vi "Camera_control_v5.vi"() -> ()   [LabVIEW 2018]
uses:
  C:/Program Files/National Instruments/LabVIEW 2018/uc480DotNet.dll
  uc480DotNet.dll
  <vilib>/MakerHub/LINX/Public/Peripherals/PWM/PWM Set Duty Cycle 1 Chan.vi
  <vilib>/MakerHub/LINX/Public/Utilities/Open Serial.vi
  <vilib>/MakerHub/LINX/Public/Peripherals/PWM/PWM Set Duty Cycle N Chans.vi
  System.Windows.Forms
  <vilib>/MakerHub/LINX/LMH-LINX.lvlib
panel:
  in  "Lamp After On (seconds)":dbl=0.5
  in  "Lamp Prior On (seconds)":dbl=0.5
  in  "Analogue out (PWM) Channel":u8=3
  in  "Serial Port":refnum<visa-resource-name>
  out "Time Stamp 5":timestamp format="%<%H:%M:%S\n%Y/%m/%d>T"
  out "Time Stamp 2":timestamp format="%<%H:%M:%S\n%Y/%m/%d>T"
  out "Boolean":bool
  out "?":u8(slide) scale=0.0..1.0
  in  "Capture Period (hours) 2":dbl=0.005
  in  "stop":bool
  out "Image":picture
  in  "Capture Frequency (minutes)":dbl=0.5
  out "Time Stamp":timestamp format="%<%H:%M:%S\n%Y/%m/%d>T"
  in  "Name of Operator":string="AT"
  in  "Parent Folder":path=path "D:/Dropbox (MIT)/Buonassisi-Group/AMD Team/Campaign 2.0/Degradation"
  in  "Zoom":u16(ring)=1 items=["4X"=4, "2X"=2, "1X"=1]
  in  "PictureBox":refnum<k24>(container)
  out "Serial Number 2":string
  out "Height 2":i32=8
  out "Width 2":i32=8
  out "Bits/Pixel 2":i32=8
  in  "Camera ID":i32
  out "Serial Number":string
  out "Height":i32=8
  out "Width":i32=8
  out "Bits/Pixel":i32=8
  in  "Pixelclock":i32(slide)=33 min=5 max=40 step=1 scale=5.0..40.0
  in  "Framerate":dbl(slide)=33.21525 min=0.47411700449083627 max=15.001275108384213 step=0.014032998230479876 scale=0.47411700449083627..15.001275108384213 scale format="%#.3g"
  in  "Exposure":dbl(slide)=33.21525 min=0.06241666666666667 max=99.86666666666667 step=0.06241666666666667 scale=0.06241666666666667..99.86666666666667 scale format="%#.3g"
  out "Error Out":errorcluster caption="error"
  in  "Load Parameter":bool
  in  "Exit Camera":bool
  in  "Stop Live":bool
  in  "Start Live":bool
  in  "Init Camera":bool
  # "Lamp Control via Arduino (LINX).\n\nSet-up Instructions\n1. Click Tools-->MakerHub-->LINX-->LINX Firmware Wizard\n2. Select Arduino type-->Next\n3. Select the COM Port associated with Arduino.\n    (can be found clicking 'Refresh' from the dropdown)-->Next\n4. Click Next\n5. Click Finish"
  # "Select the COM Port"
  # "Select the Arduino PWM pin\nto which the lamp is connected"
  # "Time for lamp to stablize before each run of photo taking"
  # "Time for lamp to stay on after each run of photo taking"
  # "This is not functional!!! Needs debugging"
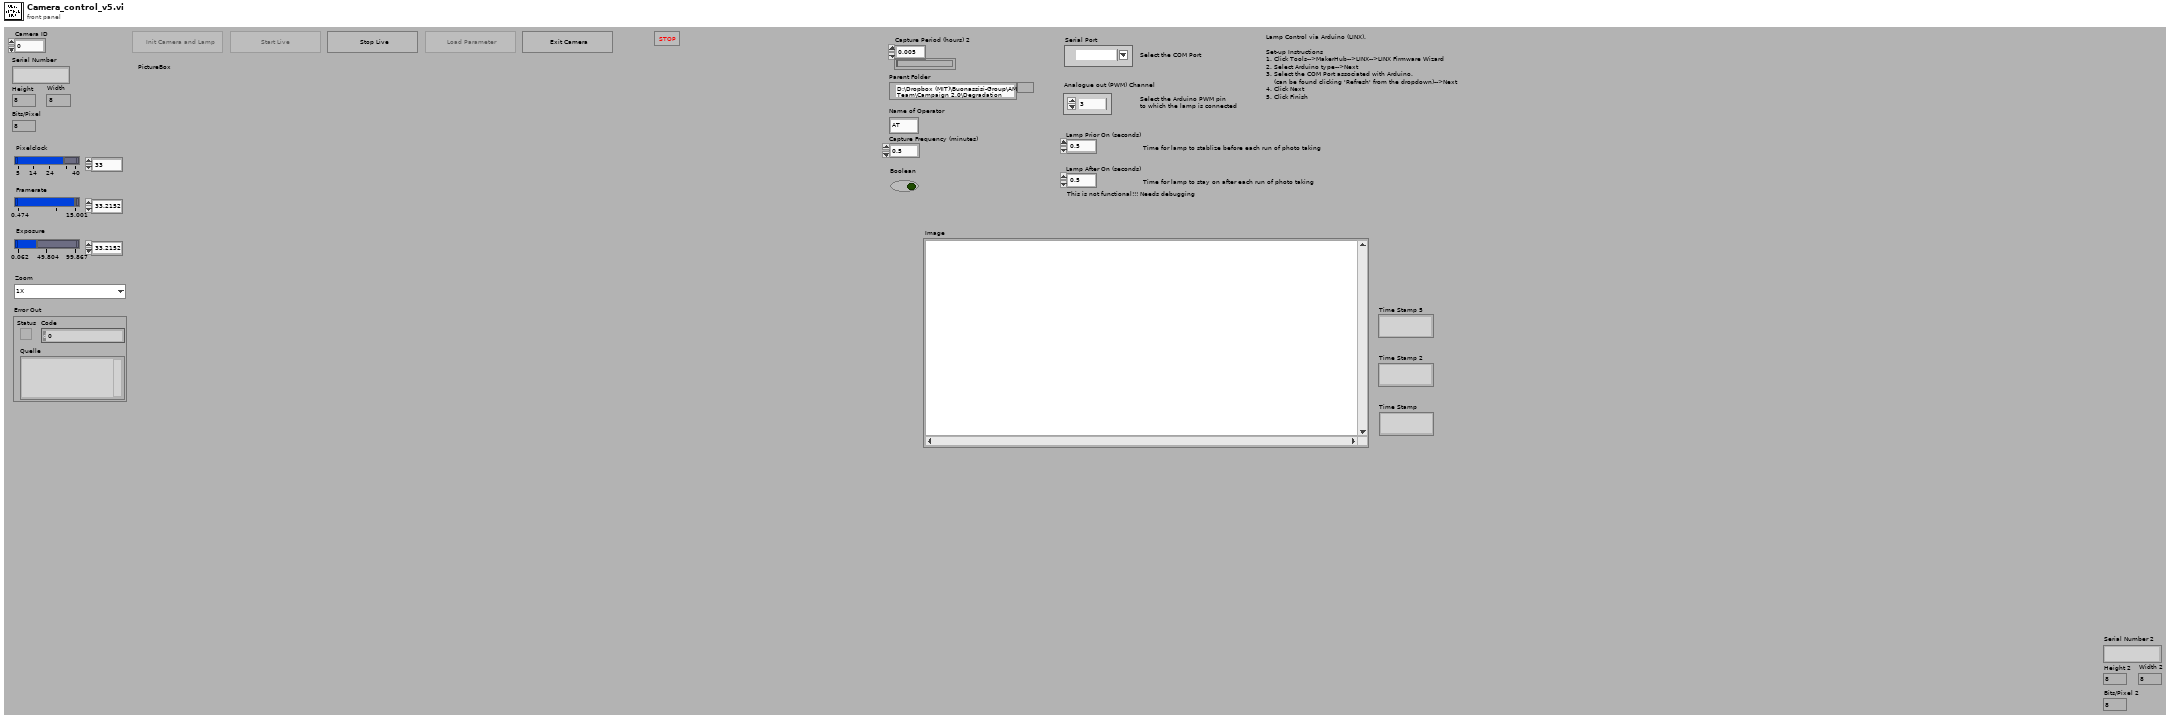
[diagram p1: front panel]
types:
  T1 = typedef "LMH-LINX.lvlib/LINX Ref.ctl" = cluster{"IO":T2, "Interface":T3, "LINX Device Config":T4}
  T2 = typedef "LMH-LINX.lvlib/Platform.ctl" = enum16{"Remote", "Local"}
  T3 = typedef "LMH-LINX.lvlib/Interface.ctl" = enum16{"Serial", "TCP"}
  T4 = typedef "LMH-LINX.lvlib/Device.lvlib/LINX Device Config.ctl" = cluster{"Interface":T3, "COM Port":refnum<visa-resource-name>, "TCP Configuration":T5, "Device Family":u8, "Device ID":u8, "Device Name":string, "TCP Ref":refnum<k5>, "Channels":T6}
  T5 = typedef "LMH-LINX.lvlib/Device.lvlib/TCP Config.ctl" = cluster{"IP Address":string, "Port":u16}
  T6 = typedef "LMH-LINX.lvlib/Channels.ctl" = cluster{"DI":u8[], "DO":u8[], "AI":u8[], "AO":u8[], "PWM":u8[], "QE":u8[], "UART":u8[], "I2C 2":u8[], "SPI":u8[], "CAN":u8[], "Servo":u8[], "AI Ref (V)":dbl, "AI Resolution (Bits)":u8, "AO Ref (V)":dbl, "AO Resolution (Bits)":u8}
  T7 = enum8{"Enabled", "Disabled", "Disabled and Grayed Out"}
  T8 = typedef "imagedata.ctl" = cluster{"image type":i32, "image depth":i32, "image":u8[], "mask":u8[], "colors":u32[], "Rectangle":cluster{"left":i16, "top":i16, "right":i16, "bottom":i16}}
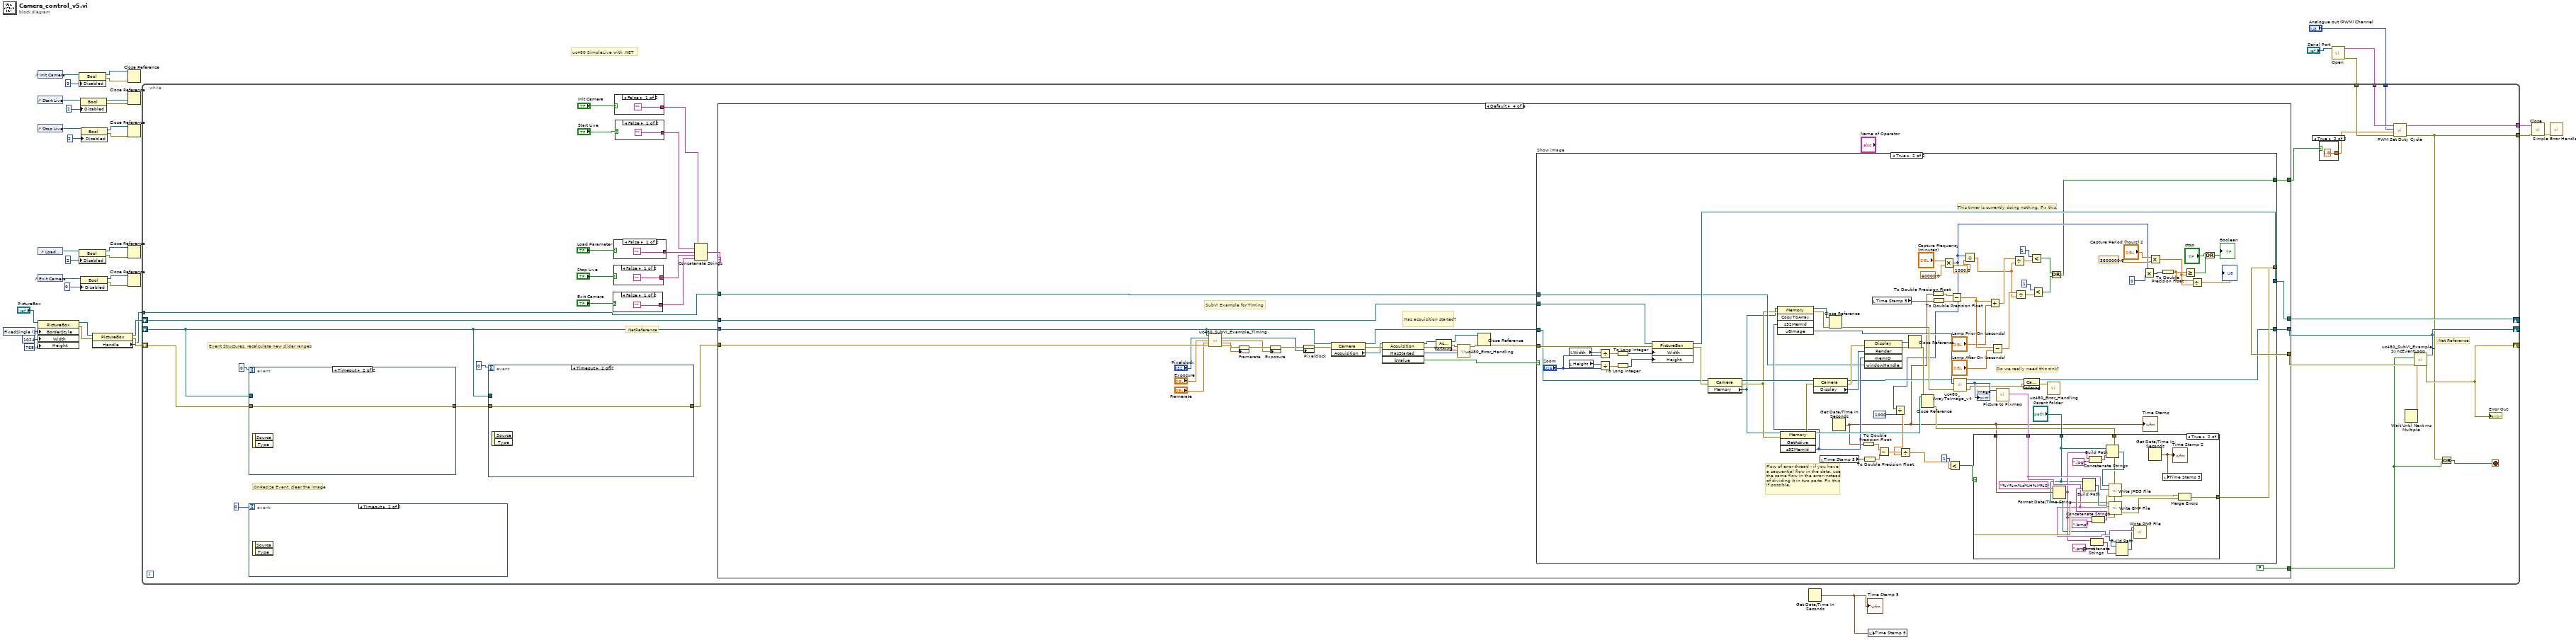
[diagram p0: block diagram]
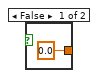
[diagram p2: hidden frame]
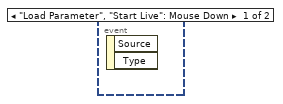
[diagram p3: hidden frame]
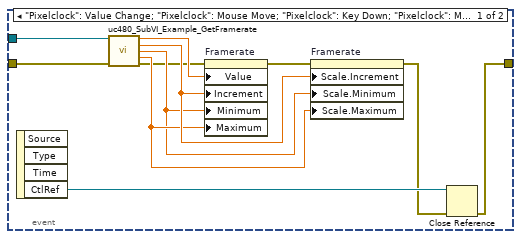
[diagram p4: hidden frame]
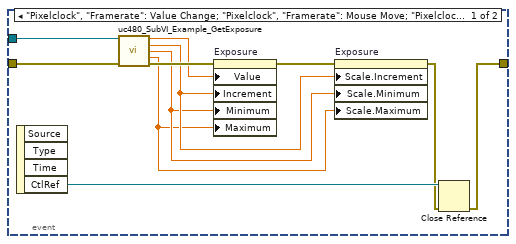
[diagram p5: hidden frame]
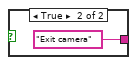
[diagram p6: hidden frame]
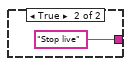
[diagram p7: hidden frame]
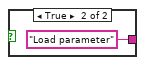
[diagram p8: hidden frame]
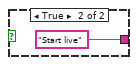
[diagram p9: hidden frame]
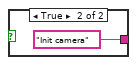
[diagram p10: hidden frame]
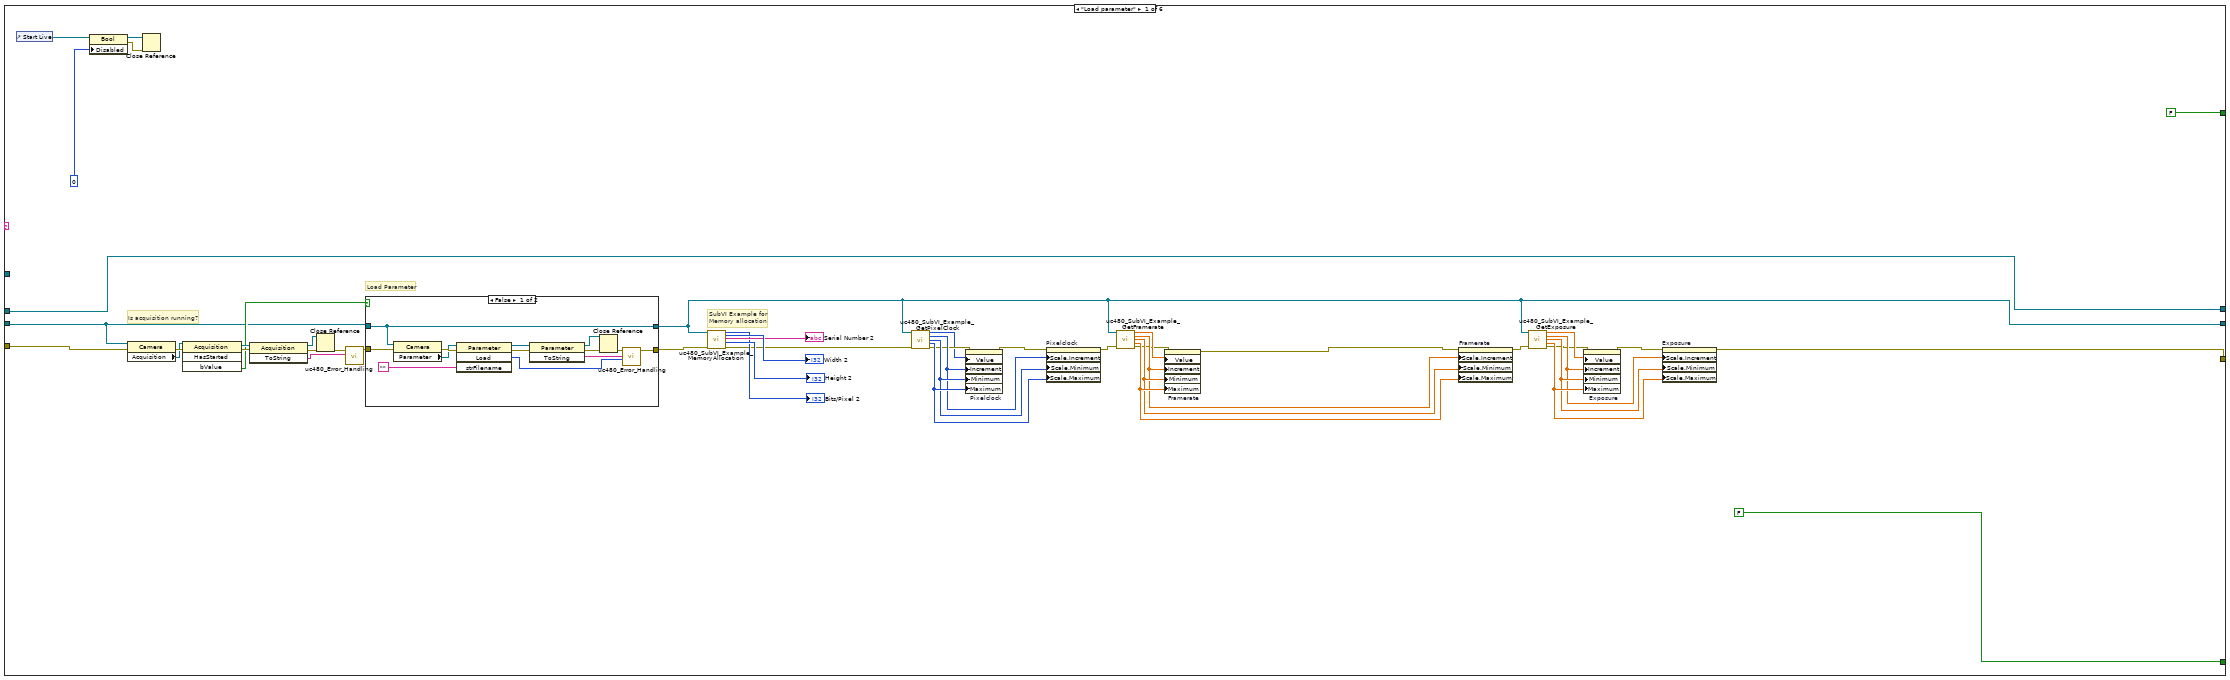
[diagram p11: hidden frame]
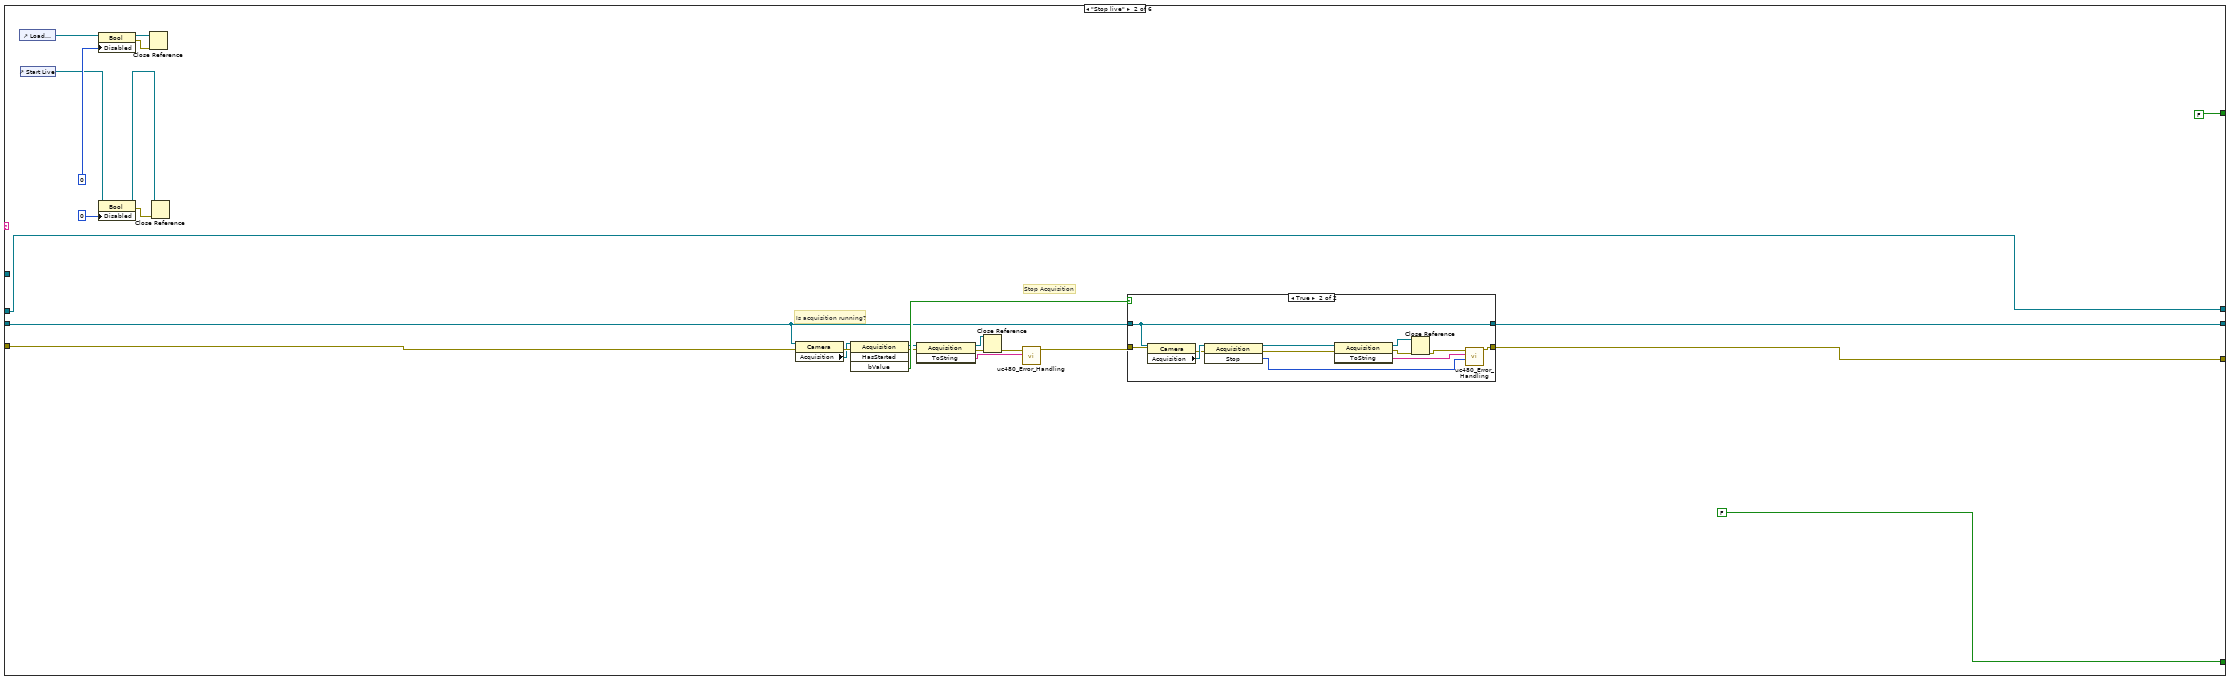
[diagram p13: hidden frame]
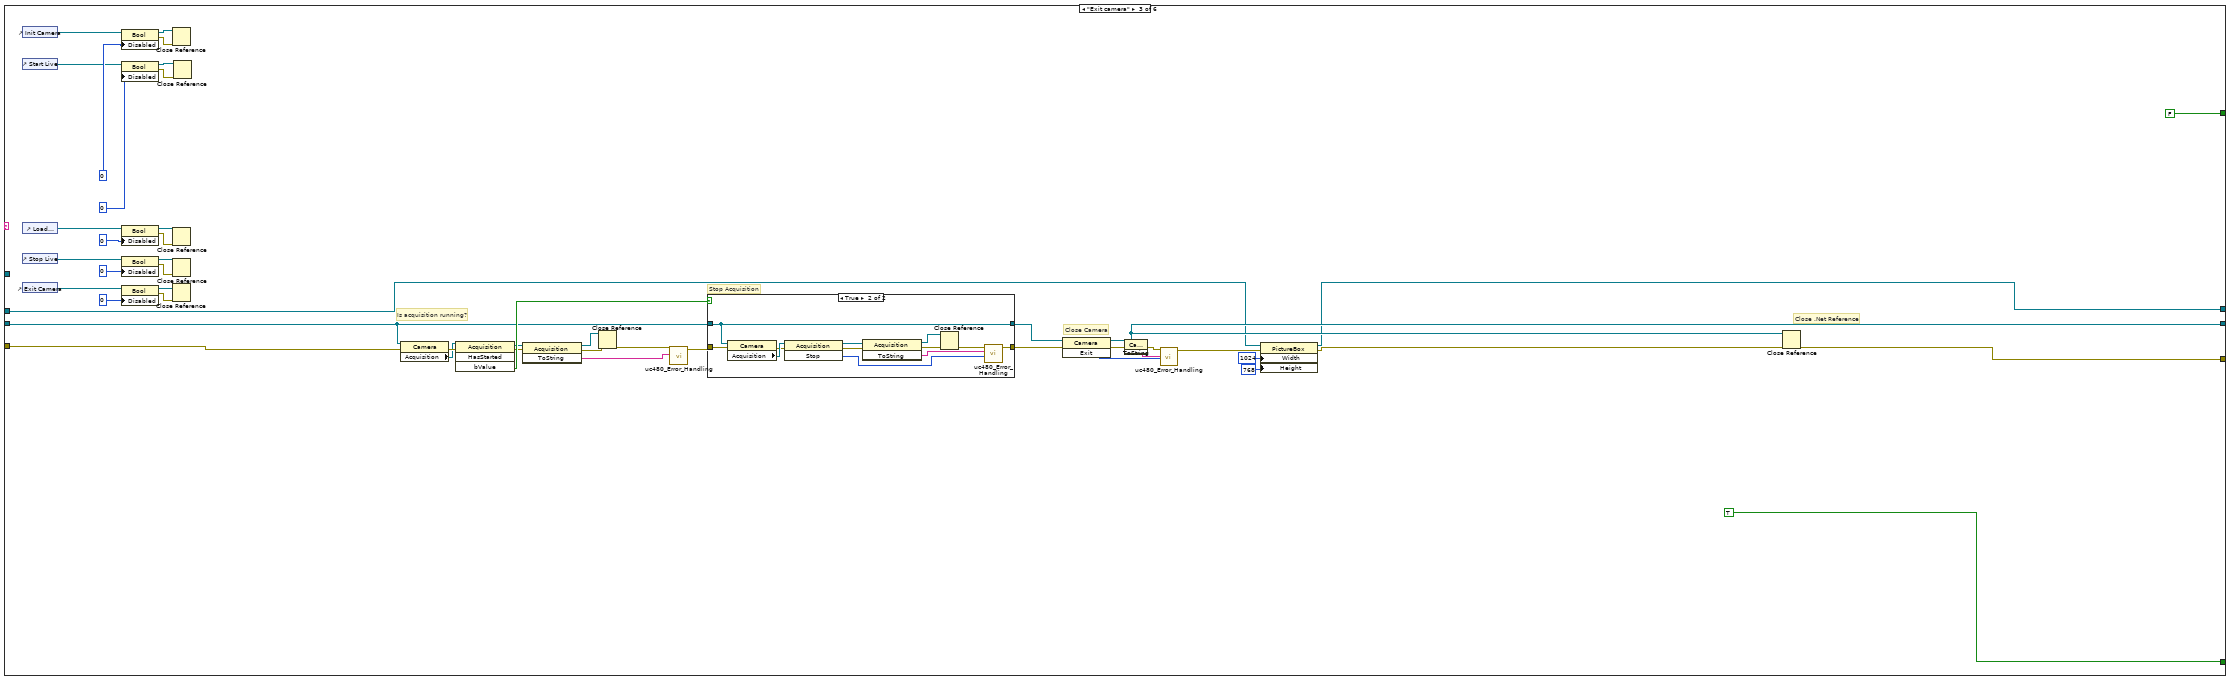
[diagram p15: hidden frame]
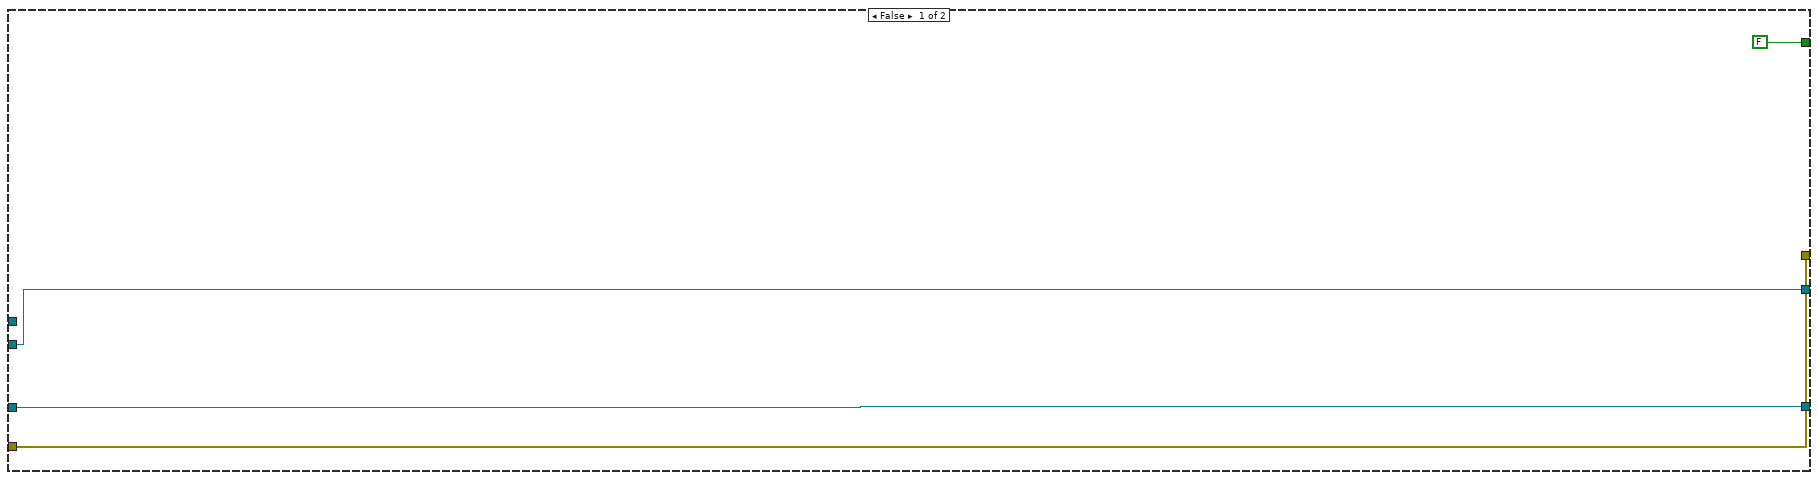
[diagram p17: hidden frame]
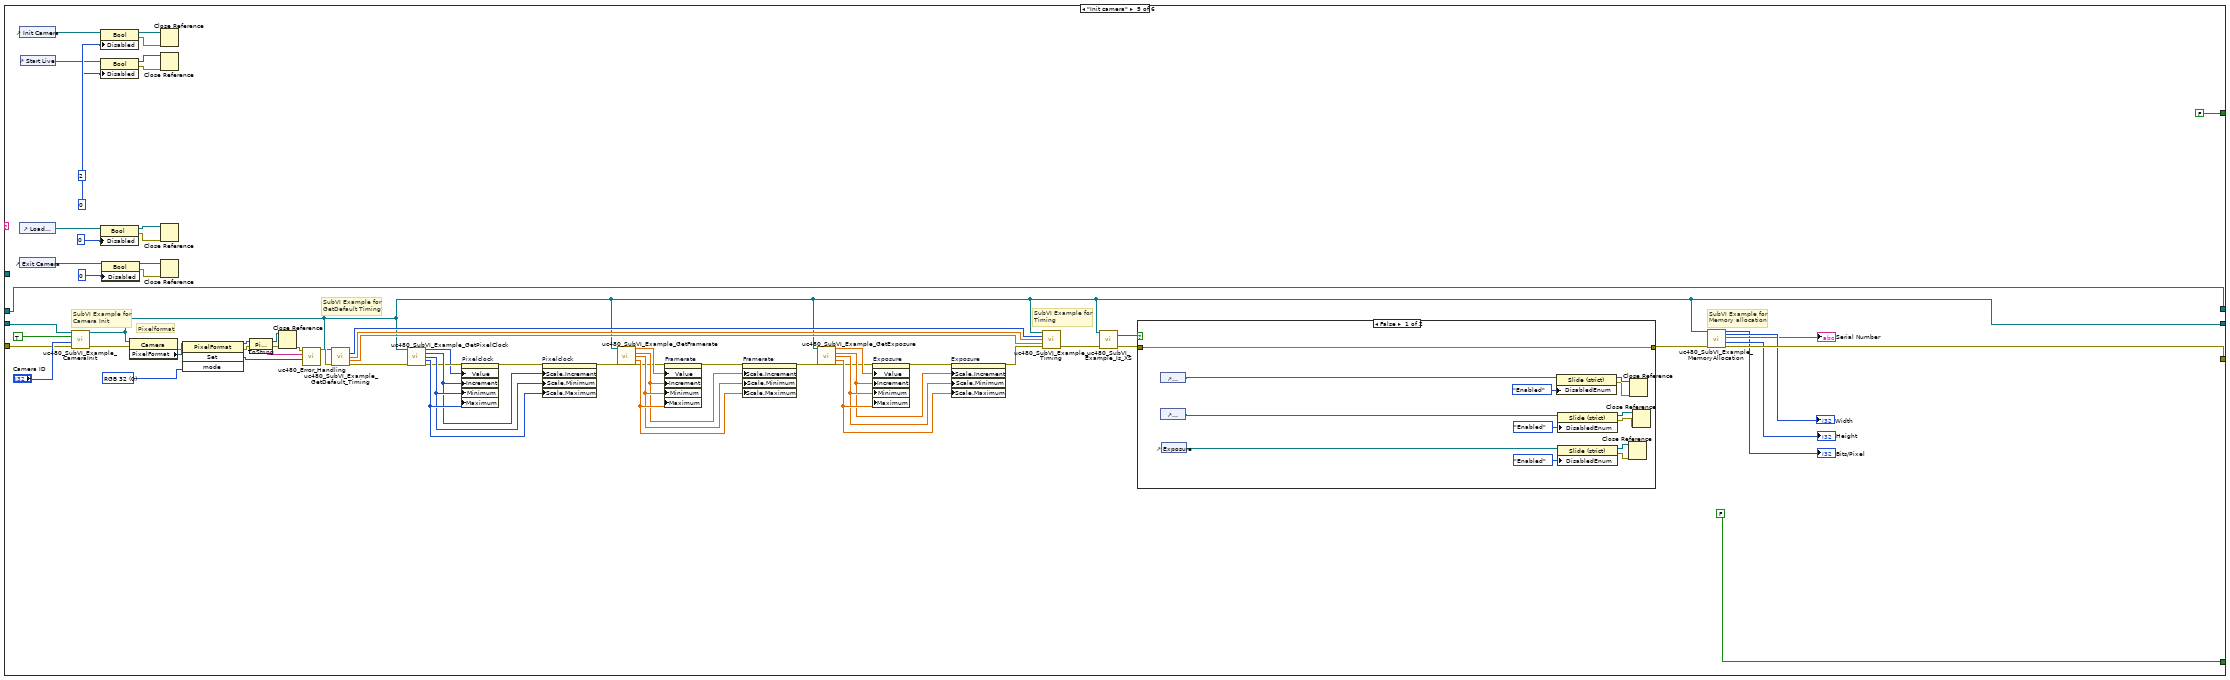
[diagram p19: hidden frame]
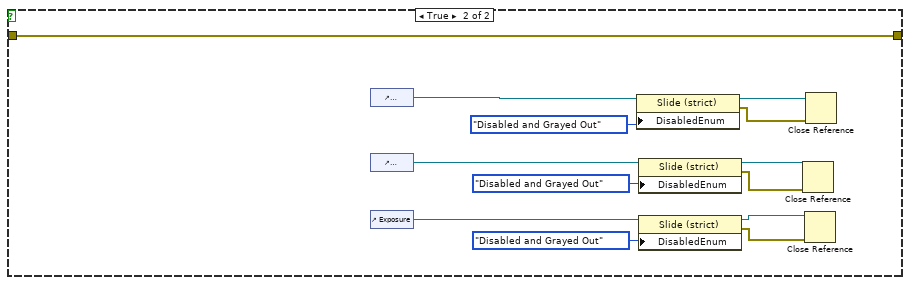
[diagram p20: hidden frame]
diagram:
  w26 = 1 items=["None", "FixedSingle", "Fixed3D"] ("BorderStyle")
  # "uc480 SimpleLive with .NET"
  n1 = control-ref of="Init Camera"() -> (w37:refnum<vi>)
  n2 = control-ref of="Start Live"() -> (w34:refnum<vi>)
  n3 = control-ref of="Stop Live"() -> (w28:refnum<vi>)
  n4 = control-ref of="Load Parameter"() -> (w29:refnum<vi>)
  n5 = control-ref of="Exit Camera"() -> (w30:refnum<vi>)
  n6 = property class="PictureBox"(reference="PictureBox", "BorderStyle"=w26, "Width"=1024, "Height"=768) -> (reference out=w12:refnum<k24>, error out=w13:errorcluster)  [unwired: 1 in]
  n7 = property class="Bool"(reference=w37, "Disabled"=u8 0 ("Deaktiviert")) -> (reference out=w23:refnum<vi>, error out=w22:errorcluster)  [unwired: 1 in]
  n8 = property class="Bool"(reference=w29, "Disabled"=u8 2 ("Deaktiviert")) -> (reference out=w17:refnum<vi>, error out=w16:errorcluster)  [unwired: 1 in]
  n9 = property class="Bool"(reference=w34, "Disabled"=u8 2 ("Deaktiviert")) -> (reference out=w21:refnum<vi>, error out=w20:errorcluster)  [unwired: 1 in]
  n10 = property class="Bool"(reference=w30, "Disabled"=u8 0 ("Deaktiviert")) -> (reference out=w15:refnum<vi>, error out=w14:errorcluster)  [unwired: 1 in]
  n11 = property class="Bool"(reference=w28, "Disabled"=u8 2 ("Deaktiviert")) -> (reference out=w19:refnum<vi>, error out=w18:errorcluster)  [unwired: 1 in]
  n12 = property class="PictureBox"(reference=w12, error in=w13) -> (reference out=w11:refnum<k24>, error out=w10:errorcluster, "Handle"=w9:refnum<k24>)
  n13 = Close Reference(reference=w23, error in (no error)=w22) -> ()  [unwired: 1 out]
  n14 = Close Reference(reference=w21, error in (no error)=w20) -> ()  [unwired: 1 out]
  n15 = Close Reference(reference=w19, error in (no error)=w18) -> ()  [unwired: 1 out]
  n16 = Close Reference(reference=w17, error in (no error)=w16) -> ()  [unwired: 1 out]
  n17 = Close Reference(reference=w15, error in (no error)=w14) -> ()  [unwired: 1 out]
  n18 = Get Date/Time In Seconds() -> (seconds since 1Jan1904=w8:timestamp)
  "Time Stamp 5" <- w8
  n19 = local write "Time Stamp 5"(w8) -> ()
  n20 = call-poly <vilib>:"Open.vi"("Serial Port"="Serial Port") -> ("Error Out"=w4:errorcluster, "LINX Resource"=w6:T1)  [unwired: 8 in, 1 out]
  n21 = while {
    shift-right: [w51] -> _
    shift-left: w10 -> [w56]
    shift-right: [w54] -> _
    shift-left: _ -> [w47]
    shift-right: [w49] -> _
    shift-left: w11 -> [w50]
    tunnel: w9 -> [w48]
    tunnel: w6 -> [w46]
    tunnel: "Analogue out (PWM) Channel" -> [w44]
    tunnel: w4 -> [w45]
    tunnel: [w41] -> w3
    tunnel: [w40] -> w2
    stop <- w42 stop-if-true
    # "OnResize Event, clear the image"
    # "Event Structures, recalculate new slider ranges"
    # ".NetReference"
    # ".Net Reference"
    n22 = event shown="[1] Timeout" {
      selector: _ -> [_ _]
      dyn-events: _ -> [_ _]
      timeout: 0 -> [_ _]
      tunnel: [w74 w85] -> w57
      tunnel: w56 -> [w84 w85]
      tunnel: w47 -> [w83 _]
      event "Pixelclock": Value Change; "Pixelclock": Mouse Move; "Pixelclock": Key Down; "Pixelclock": Mouse Up {
        n23 = event-data() -> ("CtlRef"=w76:refnum<vi>)  [unwired: 1 in, 3 out]
        n24 = call <instrlib>:"uc480_SubVI_Example_GetFramerate.vi"(".NET (Reference)"=w83, "Error In"=w84) -> ("Framerate"=w82:dbl, "Inc"=w81:dbl, "Min"=w79:dbl, "Max"=w80:dbl, "error out"=w78:errorcluster)  [unwired: 9 in]
        n25 = property on="Framerate" class="Slide (strict)"(error in=w78, "Value"=w82, "Increment"=w81, "Minimum"=w79, "Maximum"=w80) -> (error out=w77:errorcluster)  [unwired: 1 in, 1 out]
        n26 = property on="Framerate" class="Slide (strict)"(error in=w77, "Scale.Increment"=w81, "Scale.Minimum"=w79, "Scale.Maximum"=w80) -> (error out=w75:errorcluster)  [unwired: 1 in, 1 out]
        n27 = Close Reference(reference=w76, error in (no error)=w75) -> (error out=w74:errorcluster)
      }
      event Timeout {
        n28 = event-data() -> ()  [unwired: 1 in, 2 out]
      }
    }
    n29 = event shown="[1] Timeout" {
      selector: _ -> [_ _]
      dyn-events: _ -> [_ _]
      timeout: 0 -> [_ _]
      event "Load Parameter", "Start Live": Mouse Down {
        n30 = event-data() -> ()  [unwired: 1 in, 2 out]
      }
      event Timeout {
        n31 = event-data() -> ()  [unwired: 1 in, 2 out]
      }
    }
    n32 = event shown="[1] Timeout" {
      selector: _ -> [_ _]
      dyn-events: _ -> [_ _]
      timeout: 0 -> [_ _]
      tunnel: w57 -> [w96 w97]
      tunnel: [w86 w97] -> w59
      tunnel: w47 -> [w95 _]
      event "Pixelclock", "Framerate": Value Change; "Pixelclock", "Framerate": Mouse Move; "Pixelclock", "Framerate": Key Down; "Pixelclock", "Framerate": Mouse Up {
        n33 = event-data() -> ("CtlRef"=w88:refnum<vi>)  [unwired: 1 in, 3 out]
        n34 = call <instrlib>:"uc480_SubVI_Example_GetExposure.vi"(".NET (Reference)"=w95, "Error In"=w96) -> ("Exposure"=w92:dbl, "Inc"=w91:dbl, "Min"=w90:dbl, "Max"=w89:dbl, "Error out"=w93:errorcluster)  [unwired: 9 in]
        n35 = property on="Exposure" class="Slide (strict)"(error in=w93, "Value"=w92, "Increment"=w91, "Minimum"=w90, "Maximum"=w89) -> (error out=w94:errorcluster)  [unwired: 1 in, 1 out]
        n36 = property on="Exposure" class="Slide (strict)"(error in=w94, "Scale.Increment"=w91, "Scale.Minimum"=w90, "Scale.Maximum"=w89) -> (error out=w87:errorcluster)  [unwired: 1 in, 1 out]
        n37 = Close Reference(reference=w88, error in (no error)=w87) -> (error out=w86:errorcluster)
      }
      event Timeout {
        n38 = event-data() -> ()  [unwired: 1 in, 2 out]
      }
    }
    n39 = case shown="False" "Exit Camera" {
      tunnel: ["" "Exit camera"] -> w61
      frame False {
      }
      frame True {
      }
    }
    n40 = case shown="False" "Load Parameter" {
      tunnel: ["" "Load parameter"] -> w65
      frame False {
      }
      frame True {
      }
    }
    n41 = case shown="False" "Stop Live" {
      tunnel: ["" "Stop live"] -> w64
      frame False {
      }
      frame True {
      }
    }
    n42 = case shown="False" "Init Camera" {
      tunnel: ["" "Init camera"] -> w69
      frame False {
      }
      frame True {
      }
    }
    n43 = case shown="False" "Start Live" {
      tunnel: ["" "Start live"] -> w68
      frame False {
      }
      frame True {
      }
    }
    n44 = Concatenate Strings(w69, w68, w65, w64, w61) -> (w67:string)
    n45 = case shown="Default" w67 {
      tunnel: w47 -> [w145 w186 w241 w284 w465 w517]
      tunnel: w59 -> [w148 w187 w242 w294 w464 w518]
      tunnel: [w115 w185 w250 w293 w421 w516] -> w54
      tunnel: [w116 w184 w251 w292 w460 w514] -> w53
      tunnel: [FALSE FALSE TRUE FALSE FALSE FALSE] -> w43
      tunnel: w50 -> [w114 w178 w221 w276 w416 w507]
      tunnel: [w114 w178 w220 w275 w416 w507] -> w49
      tunnel: w48 -> [_ _ _ w272 _ _]
      tunnel: [FALSE FALSE FALSE w271 FALSE FALSE] -> w39
      frame "Load parameter" {
        # "SubVI Example for \nMemory allocation"
        # "Is acquisition running?"
        # "Load Parameter"
        n46 = control-ref of="Start Live"() -> (w139:refnum<vi>)
        n47 = property class="Bool"(reference=w139, "Disabled"=u8 0 ("Deaktiviert")) -> (reference out=w113:refnum<vi>, error out=w112:errorcluster)  [unwired: 1 in]
        n48 = property class="Camera"(reference=w145, error in=w148) -> (error out=w153:errorcluster, "Acquisition"=w152:refnum<k24>)  [unwired: 1 out]
        n49 = Close Reference(reference=w113, error in (no error)=w112) -> ()  [unwired: 1 out]
        n50 = invoke class="Acquisition" method="HasStarted"(reference=w152, error in=w153) -> (reference out=w149:refnum<k24>, error out=w151:errorcluster, "bValue"=w147:bool)  [unwired: 2 in, 1 out]
        n51 = invoke class="Acquisition" method="ToString"(reference=w149, error in=w151) -> (reference out=w111:refnum<k24>, error out=w110:errorcluster, "ToString"=w150:string)  [unwired: 1 in]
        n52 = Close Reference(reference=w111, error in (no error)=w110) -> (error out=w109:errorcluster)
        n53 = call <instrlib>:"uc480_Error_Handling.vi"("Error String"=w150, "Error In"=w109) -> ("Error Out"=w146:errorcluster)  [unwired: 9 in]
        n54 = case shown="False" w147 {
          tunnel: w146 -> [w161 w168]
          tunnel: w145 -> [w159 w169]
          tunnel: [w160 w168] -> w140
          tunnel: [w159 w169] -> w115
          frame False {
            n55 = property class="Camera"(reference=w159, error in=w161) -> (error out=w163:errorcluster, "Parameter"=w162:refnum<k24>)  [unwired: 1 out]
            n56 = invoke class="Parameter" method="Load"(reference=w162, error in=w163, "strFilename"="") -> (reference out=w165:refnum<k24>, error out=w166:errorcluster, "Load"=w158:i32)  [unwired: 1 in, 1 out]
            n57 = invoke class="Parameter" method="ToString"(reference=w165, error in=w166) -> (reference out=w155:refnum<k24>, error out=w157:errorcluster, "ToString"=w167:string)  [unwired: 1 in]
            n58 = Close Reference(reference=w155, error in (no error)=w157) -> (error out=w156:errorcluster)
            n59 = call <instrlib>:"uc480_Error_Handling.vi"("Error Code"=w158, "Error String"=w167, "Error In"=w156) -> ("Error Out"=w160:errorcluster)  [unwired: 8 in]
          }
          frame True {
          }
        }
        n60 = call <instrlib>:"uc480_SubVI_Example_MemoryAllocation.vi"(".NET (Reference)"=w115, "Error In"=w140) -> ("Bits/Pixel 2"=→"Bits/Pixel 2":i32, "Width"=→"Width 2":i32, "Serial Number"=→"Serial Number 2":string, "Height"=→"Height 2":i32, "Error Out"=w117:errorcluster)  [unwired: 13 in]
        n61 = call <instrlib>:"uc480_SubVI_Example_GetPixelClock.vi"(".NET (Reference)"=w115, "Error In"=w117) -> ("Pixel Clock"=w118:i32, "Inc"=w120:i32, "Min"=w121:i32, "Max"=w122:i32, "error out"=w119:errorcluster)  [unwired: 9 in]
        n62 = property on="Pixelclock" class="Slide (strict)"(error in=w119, "Value"=w118, "Increment"=w120, "Minimum"=w121, "Maximum"=w122) -> (error out=w123:errorcluster)  [unwired: 1 in, 1 out]
        n63 = property on="Pixelclock" class="Slide (strict)"(error in=w123, "Scale.Increment"=w120, "Scale.Minimum"=w121, "Scale.Maximum"=w122) -> (error out=w124:errorcluster)  [unwired: 1 in, 1 out]
        n64 = call <instrlib>:"uc480_SubVI_Example_GetFramerate.vi"(".NET (Reference)"=w115, "Error In"=w124) -> ("Framerate"=w127:dbl, "Inc"=w128:dbl, "Min"=w129:dbl, "Max"=w130:dbl, "error out"=w126:errorcluster)  [unwired: 9 in]
        n65 = property on="Framerate" class="Slide (strict)"(error in=w126, "Value"=w127, "Increment"=w128, "Minimum"=w129, "Maximum"=w130) -> (error out=w125:errorcluster)  [unwired: 1 in, 1 out]
        n66 = property on="Framerate" class="Slide (strict)"(error in=w125, "Scale.Increment"=w128, "Scale.Minimum"=w129, "Scale.Maximum"=w130) -> (error out=w131:errorcluster)  [unwired: 1 in, 1 out]
        n67 = call <instrlib>:"uc480_SubVI_Example_GetExposure.vi"(".NET (Reference)"=w115, "Error In"=w131) -> ("Exposure"=w134:dbl, "Inc"=w135:dbl, "Min"=w136:dbl, "Max"=w137:dbl, "Error out"=w132:errorcluster)  [unwired: 9 in]
        n68 = property on="Exposure" class="Slide (strict)"(error in=w132, "Value"=w134, "Increment"=w135, "Minimum"=w136, "Maximum"=w137) -> (error out=w133:errorcluster)  [unwired: 1 in, 1 out]
        n69 = property on="Exposure" class="Slide (strict)"(error in=w133, "Scale.Increment"=w135, "Scale.Minimum"=w136, "Scale.Maximum"=w137) -> (error out=w116:errorcluster)  [unwired: 1 in, 1 out]
      }
      frame "Stop live" {
        # "Is acquisition running?"
        # "Stop Acquisition"
        n70 = control-ref of="Load Parameter"() -> (w182:refnum<vi>)
        n71 = control-ref of="Start Live"() -> (w179:refnum<vi>)
        n72 = property class="Bool"(reference=w182, "Disabled"=u8 0 ("Deaktiviert")) -> (reference out=w177:refnum<vi>, error out=w176:errorcluster)  [unwired: 1 in]
        n73 = property class="Bool"(reference=w179, "Disabled"=u8 0 ("Deaktiviert")) -> (reference out=w175:refnum<vi>, error out=w174:errorcluster)  [unwired: 1 in]
        n74 = Close Reference(reference=w177, error in (no error)=w176) -> ()  [unwired: 1 out]
        n75 = Close Reference(reference=w175, error in (no error)=w174) -> ()  [unwired: 1 out]
        n76 = property class="Camera"(reference=w186, error in=w187) -> (error out=w194:errorcluster, "Acquisition"=w193:refnum<k24>)  [unwired: 1 out]
        n77 = invoke class="Acquisition" method="HasStarted"(reference=w193, error in=w194) -> (reference out=w188:refnum<k24>, error out=w190:errorcluster, "bValue"=w192:bool)  [unwired: 2 in, 1 out]
        n78 = invoke class="Acquisition" method="ToString"(reference=w188, error in=w190) -> (reference out=w171:refnum<k24>, error out=w173:errorcluster, "ToString"=w189:string)  [unwired: 1 in]
        n79 = Close Reference(reference=w171, error in (no error)=w173) -> (error out=w172:errorcluster)
        n80 = call <instrlib>:"uc480_Error_Handling.vi"("Error String"=w189, "Error In"=w172) -> ("Error Out"=w191:errorcluster)  [unwired: 9 in]
        n81 = case shown="True" w192 {
          tunnel: [w196 w207] -> w184
          tunnel: w191 -> [w196 w208]
          tunnel: w186 -> [w195 w200]
          tunnel: [w195 w200] -> w185
          frame False {
          }
          frame True {
            n82 = property class="Camera"(reference=w200, error in=w208) -> (error out=w204:errorcluster, "Acquisition"=w205:refnum<k24>)  [unwired: 1 out]
            n83 = invoke class="Acquisition" method="Stop"(reference=w205, error in=w204) -> (reference out=w202:refnum<k24>, error out=w203:errorcluster, "Stop"=w201:i32)  [unwired: 1 in]
            n84 = invoke class="Acquisition" method="ToString"(reference=w202, error in=w203) -> (reference out=w197:refnum<k24>, error out=w199:errorcluster, "ToString"=w206:string)  [unwired: 1 in]
            n85 = Close Reference(reference=w197, error in (no error)=w199) -> (error out=w198:errorcluster)
            n86 = call <instrlib>:"uc480_Error_Handling.vi"("Error Code"=w201, "Error String"=w206, "Error In"=w198) -> ("Error Out"=w207:errorcluster)  [unwired: 8 in]
          }
        }
      }
      frame "Exit camera" {
        # "Close .Net Reference"
        # "Is acquisition running?"
        # "Stop Acquisition"
        # "Close Camera"
        n87 = control-ref of="Init Camera"() -> (w233:refnum<vi>)
        n88 = control-ref of="Start Live"() -> (w232:refnum<vi>)
        n89 = control-ref of="Load Parameter"() -> (w231:refnum<vi>)
        n90 = control-ref of="Stop Live"() -> (w230:refnum<vi>)
        n91 = control-ref of="Exit Camera"() -> (w229:refnum<vi>)
        n92 = property class="Bool"(reference=w233, "Disabled"=u8 0 ("Deaktiviert")) -> (reference out=w211:refnum<vi>, error out=w210:errorcluster)  [unwired: 1 in]
        n93 = property class="Bool"(reference=w232, "Disabled"=u8 0 ("Deaktiviert")) -> (reference out=w213:refnum<vi>, error out=w212:errorcluster)  [unwired: 1 in]
        n94 = property class="Bool"(reference=w231, "Disabled"=u8 0 ("Deaktiviert")) -> (reference out=w215:refnum<vi>, error out=w214:errorcluster)  [unwired: 1 in]
        n95 = property class="Bool"(reference=w230, "Disabled"=u8 0 ("Deaktiviert")) -> (reference out=w217:refnum<vi>, error out=w216:errorcluster)  [unwired: 1 in]
        n96 = property class="Bool"(reference=w229, "Disabled"=u8 0 ("Deaktiviert")) -> (reference out=w219:refnum<vi>, error out=w218:errorcluster)  [unwired: 1 in]
        n97 = Close Reference(reference=w211, error in (no error)=w210) -> ()  [unwired: 1 out]
        n98 = Close Reference(reference=w219, error in (no error)=w218) -> ()  [unwired: 1 out]
        n99 = Close Reference(reference=w215, error in (no error)=w214) -> ()  [unwired: 1 out]
        n100 = Close Reference(reference=w217, error in (no error)=w216) -> ()  [unwired: 1 out]
        n101 = Close Reference(reference=w213, error in (no error)=w212) -> ()  [unwired: 1 out]
        n102 = property class="Camera"(reference=w241, error in=w242) -> (error out=w249:errorcluster, "Acquisition"=w248:refnum<k24>)  [unwired: 1 out]
        n103 = invoke class="Acquisition" method="HasStarted"(reference=w248, error in=w249) -> (reference out=w243:refnum<k24>, error out=w245:errorcluster, "bValue"=w247:bool)  [unwired: 2 in, 1 out]
        n104 = invoke class="Acquisition" method="ToString"(reference=w243, error in=w245) -> (reference out=w226:refnum<k24>, error out=w228:errorcluster, "ToString"=w244:string)  [unwired: 1 in]
        n105 = Close Reference ("Close Referenz")(reference=w226, error in (no error)=w228) -> (error out=w227:errorcluster)
        n106 = call <instrlib>:"uc480_Error_Handling.vi"("Error String"=w244, "Error In"=w227) -> ("Error Out"=w246:errorcluster)  [unwired: 9 in]
        n107 = case shown="True" w247 {
          tunnel: [w258 w269] -> w239
          tunnel: w246 -> [w258 w270]
          tunnel: w241 -> [w257 w262]
          tunnel: [w257 w262] -> w240
          frame False {
          }
          frame True {
            n108 = property class="Camera"(reference=w262, error in=w270) -> (error out=w266:errorcluster, "Acquisition"=w267:refnum<k24>)  [unwired: 1 out]
            n109 = invoke class="Acquisition" method="Stop"(reference=w267, error in=w266) -> (reference out=w264:refnum<k24>, error out=w265:errorcluster, "Stop"=w263:i32)  [unwired: 1 in]
            n110 = invoke class="Acquisition" method="ToString"(reference=w264, error in=w265) -> (reference out=w259:refnum<k24>, error out=w261:errorcluster, "ToString"=w268:string)  [unwired: 1 in]
            n111 = Close Reference ("Close Referenz")(reference=w259, error in (no error)=w261) -> (error out=w260:errorcluster)
            n112 = call <instrlib>:"uc480_Error_Handling.vi"("Error Code"=w263, "Error String"=w268, "Error In"=w260) -> ("Error Out"=w269:errorcluster)  [unwired: 8 in]
          }
        }
        n113 = invoke class="Camera" method="Exit"(reference=w240, error in=w239) -> (reference out=w250:refnum<k24>, error out=w253:errorcluster, "Exit"=w252:i32)  [unwired: 1 in]
        n114 = invoke class="Camera" method="ToString"(reference=w250, error in=w253) -> (error out=w254:errorcluster, "ToString"=w255:string)  [unwired: 1 in, 1 out]
        n115 = call <instrlib>:"uc480_Error_Handling.vi"("Error Code"=w252, "Error String"=w255, "Error In"=w254) -> ("Error Out"=w225:errorcluster)  [unwired: 8 in]
        n116 = property class="PictureBox"(reference=w221, error in=w225, "Width"=1024, "Height"=768) -> (reference out=w220:refnum<k24>, error out=w224:errorcluster)
        n117 = Close Reference ("Close Referenz")(reference=w250, error in (no error)=w224) -> (error out=w251:errorcluster)
      }
      frame Default {
        # "SubVI Example for Timing"
        # "Has acquisition started?"
        n118 = call <instrlib>:"uc480_SubVI_Example_Timing.vi"(".NET (Reference)"=w284, "Pixelclock"="Pixelclock", "Exposure time"="Exposure", "Framerate"="Framerate", "Error In"=w294) -> ("Pixelclock"=w287:i32, "Exposure time"=w286:dbl, "Framerate"=w285:dbl, "Error Out"=w291:errorcluster)  [unwired: 7 in]
        n119 = property on="Framerate" class="Schieber (strikt)"(error in=w291, "Scale.RngStart"=w285) -> (error out=w290:errorcluster)  [unwired: 1 in, 1 out]
        n120 = property on="Exposure" class="Schieber (strikt)"(error in=w290, "Scale.RngStart"=w286) -> (error out=w289:errorcluster)  [unwired: 1 in, 1 out]
        n121 = property on="Pixelclock" class="Schieber (strikt)"(error in=w289, "Scale.RngStart"=w287) -> (error out=w288:errorcluster)  [unwired: 1 in, 1 out]
        n122 = property class="Camera"(reference=w284, error in=w288) -> (reference out=w277:refnum<k24>, error out=w300:errorcluster, "Acquisition"=w299:refnum<k24>)
        n123 = invoke class="Acquisition" method="HasStarted"(reference=w299, error in=w300) -> (reference out=w274:refnum<k24>, error out=w296:errorcluster, "HasStarted"=w295:i32, "bValue"=w273:bool)  [unwired: 2 in]
        n124 = invoke class="Acquisition" method="ToString"(reference=w274, error in=w296) -> (reference out=w278:refnum<k24>, error out=w298:errorcluster, "ToString"=w297:string)  [unwired: 1 in]
        n125 = call <instrlib>:"uc480_Error_Handling.vi"("Error Code"=w295, "Error String"=w297, "Error In"=w298) -> ("Error Out"=w280:errorcluster)  [unwired: 8 in]
        n126 = Close Reference(reference=w278, error in (no error)=w280) -> (error out=w279:errorcluster)
        n127 = case "Show Image" shown="True" w273 {
          tunnel: [w305 w358] -> w292
          tunnel: w279 -> [w305 w379]
          tunnel: w277 -> [w304 w355]
          tunnel: [w304 w335] -> w293
          tunnel: w276 -> [w303 w380]
          tunnel: [w303 w369] -> w275
          tunnel: w272 -> [_ w363]
          tunnel: [FALSE w306] -> w271
          frame False {
          }
          frame True {
            # "This timer is currently doing nothing. Fix this."
            # "Do we really need this sink?"
            # "Flow of error thread - if you have\na sequential flow in the data, use\nthe same flow in the error instead\nof dividing it in two parts. Fix this\nif possible."
            n128 = local read "Height"() -> (w377:i32)
            n129 = local read "Width"() -> (w373:i32)
            n130 = Divide(x=w373, y="Zoom") -> (x/y=w375:dbl)
            n131 = Divide(x=w377, y="Zoom") -> (x/y=w378:dbl)
            n132 = To Long Integer(number=w375) -> (32bit integer=w374:i32)
            n133 = To Long Integer(number=w378) -> (32bit integer=w376:i32)
            n134 = property class="PictureBox"(reference=w380, error in=w379, "Width"=w374, "Height"=w376) -> (reference out=w369:refnum<k24>, error out=w364:errorcluster)
            n135 = property class="Camera"(reference=w355, error in=w364) -> (reference out=w367:refnum<k24>, error out=w357:errorcluster, "Memory"=w356:refnum<k24>)
            n136 = invoke class="Memory" method="GetActive"(reference=w356, error in=w357) -> (reference out=w366:refnum<k24>, error out=w370:errorcluster, "s32MemId"=w365:i32)  [unwired: 2 in, 1 out]
            n137 = invoke class="Memory" method="CopyToArray"(reference=w356, error in=w357, "s32MemId"=w365) -> (reference out=w361:refnum<k24>, error out=w360:errorcluster, "u8Image"=w353:u8[])  [unwired: 2 in, 2 out]
            n138 = property class="Camera"(reference=w367, error in=w370) -> (reference out=w337:refnum<k24>, error out=w381:errorcluster, "Display"=w383:refnum<k24>)
            n139 = local read "Time Stamp 5"() -> (w325:timestamp)
            n140 = Close Reference(reference=w361, error in (no error)=w360) -> (error out=w354:errorcluster)
            n141 = Get Date/Time In Seconds() -> (seconds since 1Jan1904=w322:timestamp)
            "Time Stamp" <- w322
            n142 = To Double Precision Float(number=w322) -> (double precision float=w333:dbl)
            n143 = To Double Precision Float(number=w325) -> (double precision float=w332:dbl)
            n144 = invoke class="Display" method="Render"(reference=w383, error in=w381, "memID"=w365, "windowHandle"=w363) -> (reference out=w382:refnum<k24>, error out=w362:errorcluster)  [unwired: 1 in, 3 out]
            n145 = local read "Time Stamp 5"() -> (w324:timestamp)
            n146 = Subtract(x=w333, y=w332) -> (x-y=w331:dbl)
            n147 = Close Reference(reference=w382, error in (no error)=w362) -> (error out=w371:errorcluster)
            n148 = Close Reference(reference=w366, error in (no error)=w371) -> (error out=w338:errorcluster)
            n149 = To Double Precision Float(number=w322) -> (double precision float=w321:dbl)
            n150 = To Double Precision Float(number=w324) -> (double precision float=w323:dbl)
            n151 = Multiply(x="Capture Frequency (minutes)", y=60000.0) -> (x*y=w320:i32)
            n152 = Divide(x=w320, y=1000) -> (x/y=w326:dbl)
            n153 = Divide(x=w331, y=w326) -> (x/y=w329:dbl)
            n154 = Less?(x=1, y=w329) -> (x < y?=w334:bool)
            n155 = Subtract(x=w321, y=w323) -> (x-y=w317:dbl)
            n156 = call "uc480_ArrayToImage_v4.vi"("Error In"=w354, "InArray"=w353, ".NET (Reference)"=w337) -> ("Error Out"=w341:errorcluster, "Image"=w343:picture, ".NET (Reference) 2"=w336:refnum<k24>)  [unwired: 6 in]
            "Image" <- w343
            n157 = Divide(x=w320, y=1000.0) -> (x/y=w309:dbl)
            n158 = Add(x=w317, y="Lamp Prior On (seconds)") -> (x+y=w313:dbl)
            n159 = Subtract(x=w317, y="Lamp After On (seconds)") -> (x-y=w310:dbl)
            n160 = call <vilib>:"Picture to Pixmap.vi"("picture"=w343) -> ("image data"=w344:T8)  [unwired: 9 in, 1 out]
            n161 = case shown="True" w334 {
              tunnel: "Parent Folder" -> [_ w386]
              tunnel: [w384 w403] -> w358
              tunnel: w322 -> [_ w399]
              tunnel: w344 -> [_ w390]
              tunnel: w338 -> [w384 w392]
              frame False {
              }
              frame True {
                n162 = Format Date/Time String(time format string (%c)="%Y%m%d%H%M%S", seconds (now)=w399) -> (date/time string=w388:string)  [unwired: 1 in]
                n163 = Concatenate Strings(w388, ".jpg") -> (w397:string)
                n164 = Concatenate Strings(w388, ".png") -> (w387:string)
                n165 = Concatenate Strings(w388, ".bmp") -> (w393:string)
                n166 = Build Path(base path=w386, name or relative path=w393) -> (appended path=w395:path)
                n167 = Build Path(base path=w386, name or relative path=w397) -> (appended path=w396:path)
                n168 = call <vilib>:"Write JPEG File.vi"("error in (no error)"=w392, "image data"=w390, "path to JPEG file"=w396) -> ("error out"=w400:errorcluster)  [unwired: 7 in, 1 out]
                n169 = call <vilib>:"Write BMP File.vi"("error in (no error)"=w392, "image data"=w390, "path to BMP file"=w395) -> ("error out"=w401:errorcluster)  [unwired: 7 in, 1 out]
                n170 = Build Path(base path=w386, name or relative path=w387) -> (appended path=w385:path)
                n171 = call <vilib>:"Write PNG File.vi"("image data"=w390, "path to PNG file"=w385) -> ()  [unwired: 8 in, 2 out]
                n172 = Get Date/Time In Seconds() -> (seconds since 1Jan1904=w391:timestamp)
                "Time Stamp 2" <- w391
                n173 = local write "Time Stamp 5"(w391) -> ()
                n174 = Merge Errors(w400, w401) -> (w403:errorcluster)
              }
            }
            n175 = Divide(x=w313, y=w309) -> (x/y=w312:dbl)
            n176 = Divide(x=w310, y=w309) -> (x/y=w311:dbl)
            n177 = invoke class="Camera" method="ToString"(reference=w336, error in=w341) -> (reference out=w335:refnum<k24>, error out=w342:errorcluster)  [unwired: 1 in, 1 out]
            n178 = Less?(x=1, y=w312) -> (x < y?=w307:bool)
            n179 = Less?(x=1, y=w311) -> (x < y?=w308:bool)
            n180 = call <instrlib>:"uc480_Error_Handling.vi"("Error In"=w342) -> ()  [unwired: 10 in, 1 out]
            n181 = Or(x=w307, y=w308) -> (x .or. y?=w306:bool)
            n182 = Multiply(x=w320, y=0) -> (x*y=w352:i32)
            n183 = Multiply(x="Capture Period (hours) 2", y=3600000.0) -> (x*y=w348:dbl)
            n184 = To Double Precision Float(number=w352) -> (double precision float=w349:dbl)
            n185 = Greater Or Equal?(x=w349, y=w348) -> (x >= y?=w346:bool)
            n186 = Divide(x=w349, y=w348) -> (x/y=→"?":dbl)
            n187 = Or(x="stop", y=w346) -> (x .or. y?=→"Boolean":bool)
          }
        }
      }
      frame "Init camera" {
        w473 = 0 items=["RGB 32"=0, "RGB 24"=1, "Y8 Monochrom"=6] ("Mode")
        # "SubVI Example for \nGetDefault Timing"
        # "SubVI Example for \nMemory allocation"
        # "SubVI Example for \nTiming"
        # "SubVI Example for \nCamera Init"
        # "Pixelformat"
        n188 = control-ref of="Init Camera"() -> (w428:refnum<vi>)
        n189 = control-ref of="Load Parameter"() -> (w424:refnum<vi>)
        n190 = control-ref of="Exit Camera"() -> (w422:refnum<vi>)
        n191 = control-ref of="Start Live"() -> (w426:refnum<vi>)
        n192 = call <instrlib>:"uc480_SubVI_Example_CameraInit.vi"("Error In"=w464, "Camera ID"="Camera ID", "Init Camera Flag"=TRUE, ".NET (Reference)"=w465) -> ("Error Out"=w470:errorcluster, ".NET (Reference)"=w421:refnum<k24>)  [unwired: 6 in]
        n193 = property class="Bool"(reference=w424, "Disabled"=u8 0 ("Deaktiviert")) -> (reference out=w411:refnum<vi>, error out=w410:errorcluster)  [unwired: 1 in]
        n194 = property class="Bool"(reference=w428, "Disabled"=u8 2 ("Deaktiviert")) -> (reference out=w415:refnum<vi>, error out=w414:errorcluster)  [unwired: 1 in]
        n195 = property class="Bool"(reference=w426, "Disabled"=u8 0 ("Deaktiviert")) -> (reference out=w413:refnum<vi>, error out=w412:errorcluster)  [unwired: 1 in]
        n196 = property class="Bool"(reference=w422, "Disabled"=u8 0 ("Deaktiviert")) -> (reference out=w409:refnum<vi>, error out=w408:errorcluster)  [unwired: 1 in]
        n197 = property on="Property Node" class="Camera"(reference=w421, error in=w470) -> (error out=w471:errorcluster, "PixelFormat"=w472:refnum<k24>)  [unwired: 1 out]
        n198 = Close Reference(reference=w415, error in (no error)=w414) -> ()  [unwired: 1 out]
        n199 = Close Reference(reference=w413, error in (no error)=w412) -> ()  [unwired: 1 out]
        n200 = Close Reference(reference=w411, error in (no error)=w410) -> ()  [unwired: 1 out]
        n201 = Close Reference(reference=w409, error in (no error)=w408) -> ()  [unwired: 1 out]
        n202 = invoke class="PixelFormat" method="Set"(reference=w472, error in=w471, "mode"=w473) -> (reference out=w468:refnum<k24>, error out=w461:errorcluster, "Set"=w467:i32)  [unwired: 1 in, 1 out]
        n203 = invoke class="PixelFormat" method="ToString"(reference=w468, error in=w461) -> (reference out=w405:refnum<k24>, error out=w407:errorcluster, "ToString"=w469:string)  [unwired: 1 in]
        n204 = Close Reference(reference=w405, error in (no error)=w407) -> (error out=w406:errorcluster)
        n205 = call <instrlib>:"uc480_Error_Handling.vi"("Error Code"=w467, "Error String"=w469, "Error In"=w406) -> ("Error Out"=w435:errorcluster)  [unwired: 8 in]
        n206 = call <instrlib>:"uc480_SubVI_Example_GetDefault_Timing.vi"(".NET (Reference)"=w421, "Error In"=w435) -> ("Pixelclock"=w434:i32, "Exposure time"=w433:dbl, "Framerate"=w432:dbl, "Error Out"=w431:errorcluster)  [unwired: 10 in]
        n207 = call <instrlib>:"uc480_SubVI_Example_GetPixelClock.vi"(".NET (Reference)"=w421, "Error In"=w431) -> ("Pixel Clock"=w436:i32, "Inc"=w438:i32, "Min"=w439:i32, "Max"=w440:i32, "error out"=w437:errorcluster)  [unwired: 9 in]
        n208 = property on="Pixelclock" class="Slide (strict)"(error in=w437, "Value"=w436, "Increment"=w438, "Minimum"=w439, "Maximum"=w440) -> (error out=w441:errorcluster)  [unwired: 1 in, 1 out]
        n209 = property on="Pixelclock" class="Slide (strict)"(error in=w441, "Scale.Increment"=w438, "Scale.Minimum"=w439, "Scale.Maximum"=w440) -> (error out=w442:errorcluster)  [unwired: 1 in, 1 out]
        n210 = call <instrlib>:"uc480_SubVI_Example_GetFramerate.vi"(".NET (Reference)"=w421, "Error In"=w442) -> ("Framerate"=w445:dbl, "Inc"=w446:dbl, "Min"=w447:dbl, "Max"=w448:dbl, "error out"=w444:errorcluster)  [unwired: 9 in]
        n211 = property on="Framerate" class="Slide (strict)"(error in=w444, "Value"=w445, "Increment"=w446, "Minimum"=w447, "Maximum"=w448) -> (error out=w443:errorcluster)  [unwired: 1 in, 1 out]
        n212 = property on="Framerate" class="Slide (strict)"(error in=w443, "Scale.Increment"=w446, "Scale.Minimum"=w447, "Scale.Maximum"=w448) -> (error out=w449:errorcluster)  [unwired: 1 in, 1 out]
        n213 = call <instrlib>:"uc480_SubVI_Example_GetExposure.vi"(".NET (Reference)"=w421, "Error In"=w449) -> ("Exposure"=w452:dbl, "Inc"=w453:dbl, "Min"=w454:dbl, "Max"=w455:dbl, "Error out"=w450:errorcluster)  [unwired: 9 in]
        n214 = property on="Exposure" class="Slide (strict)"(error in=w450, "Value"=w452, "Increment"=w453, "Minimum"=w454, "Maximum"=w455) -> (error out=w451:errorcluster)  [unwired: 1 in, 1 out]
        n215 = property on="Exposure" class="Slide (strict)"(error in=w451, "Scale.Increment"=w453, "Scale.Minimum"=w454, "Scale.Maximum"=w455) -> (error out=w430:errorcluster)  [unwired: 1 in, 1 out]
        n216 = call <instrlib>:"uc480_SubVI_Example_Timing.vi"(".NET (Reference)"=w421, "Pixelclock"=w434, "Exposure time"=w433, "Framerate"=w432, "Error In"=w430) -> ("Error Out"=w420:errorcluster)  [unwired: 7 in, 3 out]
        n217 = call <instrlib>:"uc480_SubVI_Example_Is_XS.vi"("Error In"=w420, ".NET (Reference)"=w421) -> ("Error Out"=w417:errorcluster, "IsXS"=w419:bool)  [unwired: 7 in, 1 out]
        n218 = case shown="False" w419 {
          tunnel: w417 -> [w486 w499]
          tunnel: [w486 w499] -> w418
          frame False {
            n219 = control-ref of="Pixelclock"() -> (w482:refnum<vi>)
            n220 = control-ref of="Framerate"() -> (w481:refnum<vi>)
            n221 = control-ref of="Exposure"() -> (w480:refnum<vi>)
            n222 = property class="Slide (strict)"(reference=w482, "DisabledEnum"=T7."Enabled" ("Disabled")) -> (reference out=w479:refnum<vi>, error out=w478:errorcluster)  [unwired: 1 in]
            n223 = property class="Slide (strict)"(reference=w481, "DisabledEnum"=T7."Enabled" ("Disabled")) -> (reference out=w477:refnum<vi>, error out=w476:errorcluster)  [unwired: 1 in]
            n224 = property class="Slide (strict)"(reference=w480, "DisabledEnum"=T7."Enabled" ("Disabled")) -> (reference out=w475:refnum<vi>, error out=w474:errorcluster)  [unwired: 1 in]
            n225 = Close Reference(reference=w475, error in (no error)=w474) -> ()  [unwired: 1 out]
            n226 = Close Reference(reference=w479, error in (no error)=w478) -> ()  [unwired: 1 out]
            n227 = Close Reference(reference=w477, error in (no error)=w476) -> ()  [unwired: 1 out]
          }
          frame True {
            n228 = control-ref of="Pixelclock"() -> (w498:refnum<vi>)
            n229 = control-ref of="Framerate"() -> (w495:refnum<vi>)
            n230 = control-ref of="Exposure"() -> (w493:refnum<vi>)
            n231 = property class="Slide (strict)"(reference=w498, "DisabledEnum"=T7."Disabled and Grayed Out" ("Disabled")) -> (reference out=w491:refnum<vi>, error out=w492:errorcluster)  [unwired: 1 in]
            n232 = property class="Slide (strict)"(reference=w495, "DisabledEnum"=T7."Disabled and Grayed Out" ("Disabled")) -> (reference out=w490:refnum<vi>, error out=w489:errorcluster)  [unwired: 1 in]
            n233 = property class="Slide (strict)"(reference=w493, "DisabledEnum"=T7."Disabled and Grayed Out" ("Disabled")) -> (reference out=w488:refnum<vi>, error out=w487:errorcluster)  [unwired: 1 in]
            n234 = Close Reference(reference=w490, error in (no error)=w489) -> ()  [unwired: 1 out]
            n235 = Close Reference(reference=w488, error in (no error)=w487) -> ()  [unwired: 1 out]
            n236 = Close Reference(reference=w491, error in (no error)=w492) -> ()  [unwired: 1 out]
          }
        }
        n237 = call <instrlib>:"uc480_SubVI_Example_MemoryAllocation.vi"(".NET (Reference)"=w421, "Error In"=w418) -> ("Bits/Pixel 2"=→"Bits/Pixel":i32, "Width"=→"Width":i32, "Serial Number"=→"Serial Number":string, "Height"=→"Height":i32, "Error Out"=w460:errorcluster)  [unwired: 13 in]
      }
      frame "Start live" {
        # "Has acquisition started?"
        # "Start Acquisition"
        n238 = control-ref of="Start Live"() -> (w513:refnum<vi>)
        n239 = control-ref of="Load Parameter"() -> (w510:refnum<vi>)
        n240 = control-ref of="Stop Live"() -> (w508:refnum<vi>)
        n241 = property class="Bool"(reference=w513, "Disabled"=u8 2 ("Deaktiviert")) -> (reference out=w502:refnum<vi>, error out=w501:errorcluster)  [unwired: 1 in]
        n242 = property class="Bool"(reference=w510, "Disabled"=u8 2 ("Deaktiviert")) -> (reference out=w504:refnum<vi>, error out=w503:errorcluster)  [unwired: 1 in]
        n243 = property class="Bool"(reference=w508, "Disabled"=u8 0 ("Deaktiviert")) -> (reference out=w506:refnum<vi>, error out=w505:errorcluster)  [unwired: 1 in]
        n244 = Close Reference(reference=w504, error in (no error)=w503) -> ()  [unwired: 1 out]
        n245 = Close Reference(reference=w502, error in (no error)=w501) -> ()  [unwired: 1 out]
        n246 = Close Reference(reference=w506, error in (no error)=w505) -> ()  [unwired: 1 out]
        n247 = property class="Camera"(reference=w517, error in=w518) -> (error out=w527:errorcluster, "Acquisition"=w526:refnum<k24>)  [unwired: 1 out]
        n248 = invoke class="Acquisition" method="HasStarted"(reference=w526, error in=w527) -> (reference out=w522:refnum<k24>, error out=w521:errorcluster, "HasStarted"=w520:i32, "bValue"=w525:bool)  [unwired: 2 in]
        n249 = invoke class="Acquisition" method="ToString"(reference=w522, error in=w521) -> (error out=w524:errorcluster, "ToString"=w523:string)  [unwired: 1 in, 1 out]
        n250 = call <instrlib>:"uc480_Error_Handling.vi"("Error Code"=w520, "Error String"=w523, "Error In"=w524) -> ("Error Out"=w519:errorcluster)  [unwired: 8 in]
        n251 = case shown="True" w525 {
          tunnel: [w530 w540] -> w514
          tunnel: w519 -> [w536 w540]
          tunnel: w517 -> [w535 w539]
          tunnel: [w535 w539] -> w516
          frame False {
            w528 = 1 items=["IS_DONT_WAIT", "IS_WAIT"] ("Wait")
            n252 = property class="Camera"(reference=w535, error in=w536) -> (error out=w537:errorcluster, "Acquisition"=w538:refnum<k24>)  [unwired: 1 out]
            n253 = invoke class="Acquisition" method="Capture"(reference=w538, error in=w537, "param"=w528) -> (reference out=w531:refnum<k24>, error out=w532:errorcluster, "Capture"=w529:i32)  [unwired: 1 in, 1 out]
            n254 = invoke class="Acquisition" method="ToString"(reference=w531, error in=w532) -> (error out=w534:errorcluster, "ToString"=w533:string)  [unwired: 1 in, 1 out]
            n255 = call <instrlib>:"uc480_Error_Handling.vi"("Error Code"=w529, "Error String"=w533, "Error In"=w534) -> ("Error Out"=w530:errorcluster)  [unwired: 8 in]
          }
          frame True {
          }
        }
      }
    }
    n256 = case shown="True" w39 {
      tunnel: [0.0 1.0 ("Duty Cycle (0-1)")] -> w38
      frame False {
      }
      frame True {
      }
    }
    n257 = call-poly <vilib>:"PWM Set Duty Cycle.vi"("Error In"=w45, "Duty Cycle (0-1)"=w38, "PWM Channel"=w44, "LINX Resource"=w46) -> ("Error Out"=w40:errorcluster, "LINX Resource"=w41:T1)  [unwired: 6 in]
    n258 = call <instrlib>:"uc480_SubVI_Example_SyncEventLoop.vi"("Error In"=w53, "use sync"=w43, ".NET (Reference)"=w54) -> ("Error Out"=w51:errorcluster, "Synchronize (ms)"=w52:dbl)  [unwired: 7 in]
    "Error Out" <- w51
    n259 = Wait Until Next ms Multiple(millisecond multiple=w52) -> ()  [unwired: 1 out]
    n260 = Or(x=w40, y=w43) -> (x .or. y?=w42:bool)
  }
  n261 = call <vilib>:"Close.vi"("Error In"=w2, "LINX Resource"=w3) -> ("Error Out"=w1:errorcluster)  [unwired: 9 in]
  n262 = call <vilib>:"Simple Error Handler.vi"("error in (no error)"=w1) -> ()  [unwired: 4 in, 5 out]
